vi "ElectrometerReadingVar.vi"() -> ()   [LabVIEW 2016]
panel:
  out "Electrometer1Reading":bool
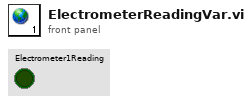
[diagram p1: front panel]
diagram:
